vi "AerotechWaitForInposition.vi"(8 "error in (no error)":errorcluster) -> (0 "error out":errorcluster)   [LabVIEW 2009]
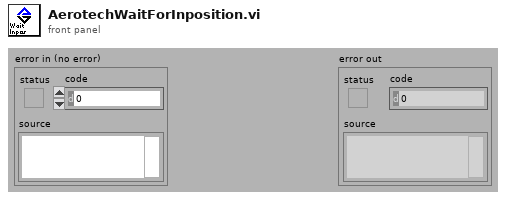
[diagram p1: front panel]
types:
  T1 = cluster{"Axis 1 active":bool, "Axis 2 active":bool, "Axis 3 active":bool, "Axis 4 active":bool, "Axis 1 not in position":bool, "Axis 2 not in position":bool, "Axis 3 not in position":bool, "Axis 4 not in position":bool, "Plane 1 comm. busy":bool, "Plane 2 comm. busy":bool, "Plane 4 comm. busy":bool, "Plane 3 comm. busy":bool, "Queue 1 buffer not empty":bool, "Queue 2 buffer not empty":bool, "Queue 3 buffer not empty":bool, "Queue 4 buffer not empty":bool, "Plane 1 halted":bool, "Plane 2 halted":bool, "Plane 3 halted":bool, "Plane 4 halted":bool, "Global abort active":bool, "Feedhold active":bool, "PC Bus Interrupt high":bool, "Not ready for next command":bool}
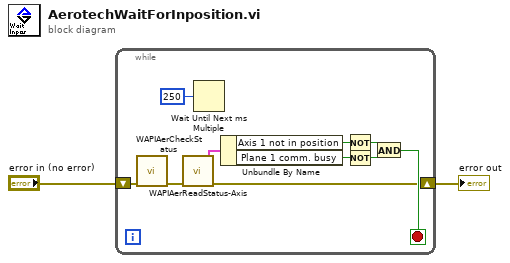
[diagram p0: block diagram]
diagram:
  n1 = while {
    shift-right: [w6] -> w1
    shift-left: "error in (no error)" -> [w8]
    stop <- w7 stop-if-true
    n2 = call "WAPIAerCheckStatus.vi"("error in (no error)"=w8) -> ("error out"=w12:errorcluster)  [unwired: 8 in]
    n3 = call "WAPIAerReadStatus-Axis.vi"("error in (no error)"=w12) -> ("Axis/Plane/Queue status"=w11:T1, "error out"=w6:errorcluster)  [unwired: 7 in]
    n4 = Wait Until Next ms Multiple(millisecond multiple=u32 250) -> ()  [unwired: 1 out]
    n5 = Unbundle By Name(w11) -> ("Axis 1 not in position"=w10:bool, "Plane 1 comm. busy"=w9:bool)
    n6 = Not(x=w10) -> (.not. x?=w4:bool)
    n7 = Not(x=w9) -> (.not. x?=w3:bool)
    n8 = And(x=w4, y=w3) -> (x .and. y?=w7:bool)
  }
  "error out" <- w1
